vi "Initialize MeasurementLink Session.vi"(7 "remote connection options":T2, 8 "error in":errorcluster, 9 "initialize and close session behavior":T1, 10 "session initialization parameters":T3, 11 "session factory in":refnum<class "Session Factory.lvclass">) -> (0 "error out":errorcluster, 2 "session out":variant, 3 "session factory out":refnum<class "Session Factory.lvclass">)   [LabVIEW 2020, in "MeasurementLink niDigital.lvlib" / "Session Factory.lvclass"]
uses:
  Session Factory.lvclass
  MeasurementLink Instrument/ISession Factory/Session Initialization Parameters.ctl
  MeasurementLink Instrument/ISession Factory/Remote Connection Options.ctl
  MeasurementLink Instrument/ISession Factory/Initialize and Close Session Behavior.ctl
  Session Factory.lvclass/Session Factory.ctl
  MeasurementLink Instrument/ISession Factory/ISession Factory.lvclass
  <instrlib>/niDigital/niDigital.llb/niDigital Initialize for gRPC Session.vi
  <instrlib>/niDigital/niDigital.llb/niDigital Attach gRPC Session.vi
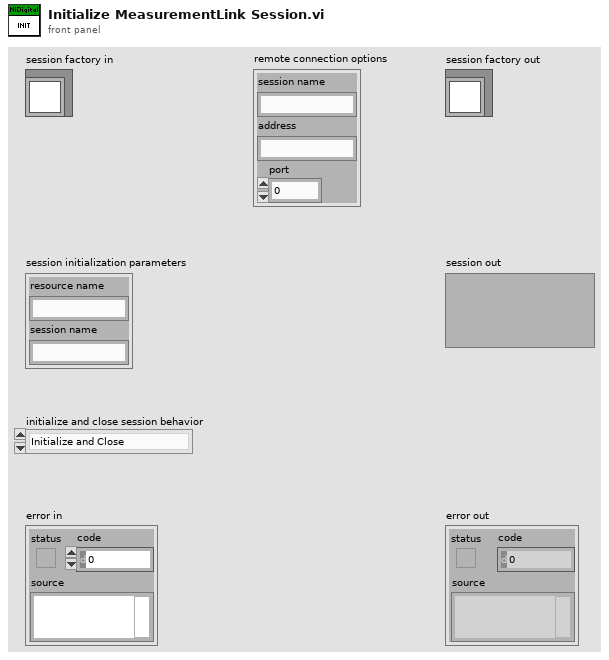
[diagram p1: front panel]
types:
  T1 = typedef "MeasurementLink Instrument.lvlib/ISession Factory.lvclass/Initialize and Close Session Behavior.ctl" = enum16{"Initialize and Close", "Attach and Detach", "Initialize and Detach", "Attach and Close"}
  T2 = typedef "MeasurementLink Instrument.lvlib/ISession Factory.lvclass/Remote Connection Options.ctl" = cluster{"session name":string, "address":string, "port":u32}
  T3 = typedef "MeasurementLink Instrument.lvlib/ISession Factory.lvclass/Session Initialization Parameters.ctl" = cluster{"resource name":string, "session name":string}
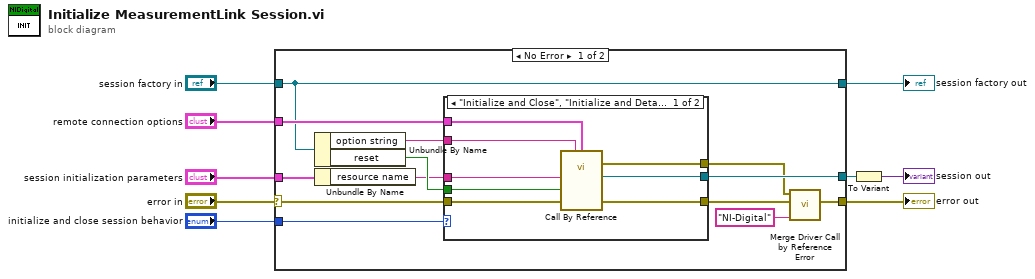
[diagram p0: block diagram]
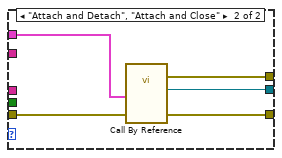
[diagram p2: hidden frame]
diagram:
  n1 = case shown="No Error" "error in" {
    selector: "error in" -> [w19 w36]
    tunnel: [w12 w36] -> w8
    tunnel: "session factory in" -> [w17 w37]
    tunnel: [w17 w37] -> w6
    tunnel: "initialize and close session behavior" -> [w22 _]
    tunnel: "remote connection options" -> [w21 _]
    tunnel: "session initialization parameters" -> [w18 _]
    tunnel: [w20 _] -> w2
    frame No Error {
      n2 = Unbundle By Name(w17) -> ("option string"=w16:string, "reset"=w15:bool)
      n3 = Unbundle By Name(w18) -> ("resource name"=w14:string)
      n4 = case shown="\"Initialize and Close\", \"Initialize and Detach\"" w22 {
        tunnel: w21 -> [w29 w35]
        tunnel: [w28 w34] -> w20
        tunnel: w19 -> [w30 w33]
        tunnel: [w27 w32] -> w13
        tunnel: w14 -> [w26 _]
        tunnel: w16 -> [w25 _]
        tunnel: w15 -> [w24 _]
        tunnel: [w23 w31] -> w11
        frame "Initialize and Close", "Initialize and Detach" {
          n5 = call-by-ref "?"("resource name"=w26, "option string"=w25, "gRPC options"=w29, "reset (F)"=w24, "error in"=w30) -> (error out=w23:errorcluster, "instrument handle"=w28:refnum<k15>, 15:"error out"=w27:errorcluster)  [unwired: 11 in, 1 out]
        }
        frame "Attach and Detach", "Attach and Close" {
          n6 = call-by-ref "?"("gRPC options"=w35, "error in"=w33) -> (error out=w31:errorcluster, "instrument handle out"=w34:refnum<k15>, 15:"error out"=w32:errorcluster)  [unwired: 14 in, 1 out]
        }
      }
      n7 = call "Merge Driver Call by Reference Error.vi"("driver name"="NI-Digital", "called vi error"=w13, "call by ref error"=w11) -> ("error out"=w12:errorcluster)  [unwired: 8 in]
    }
    frame Error {
    }
  }
  "error out" <- w8
  "session factory out" <- w6
  n8 = To Variant(anything=w2) -> (Variant=→"session out":variant)
